vi "MM9.InitDelays.vi"(0 "i ref in":refnum<vi>, 2 "InitObjs":string[](array[string]), 3 "ms timeout (10000)":i32=10000, 5 "error in (no error)":errorcluster) -> (14 "i ref out":refnum<vi>, 16 "InitObjs out":string[](array[string]), 17 "timed out":bool, 19 "error out":errorcluster)   [LabVIEW 2014, in "MM9.lvlib"]
doc: "Initializes the delays."
uses:
  MM9.lvlib
  CSCore/CSSystem/CoreDefs/CoreDefs.call_type.ctl
  CSCore/BaseProcess/BaseProcess.descriptor string definition.ctl
  CSCore/CSSystem/CoreDefs/CoreDefs.rawDataType.ctl
  CSCore/CSSystem/CoreLib/CoreLib.double 2 byte array.vi
  CSCore/BaseProcess/BaseProcess.lvlib
  LEBITLib/LEBITLib.lvlib
  CSCore/CSSystem/CoreLib/CoreLib.lvlib
panel:
  in  "CallClusterTyp":T1={"Object"="", "Selector"="", "CallType"=enum."synchronous", "Async Object"="", "Async Selector"="", "Data Descriptor"="", "Data"=[], "Error #"=0, "Expire"=0}
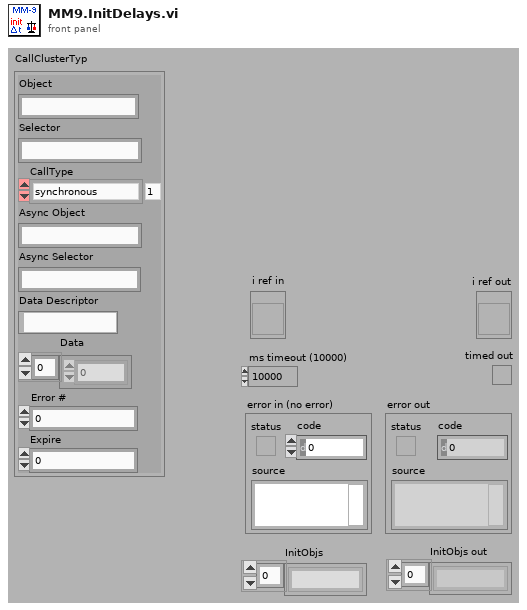
[diagram p1: front panel]
types:
  T1 = typedef "CoreDefs.call_type.ctl" = cluster{"Object":string, "Selector":string, "CallType":enum16{"simple", "synchronous", "asynchronous"}, "Async Object":string, "Async Selector":string, "Data Descriptor":T2, "Data":T3, "Error #":i32, "Expire":u32}
  T2 = typedef "BaseProcess.lvlib/BaseProcess.descriptor string definition.ctl" = string
  T3 = typedef "CoreDefs.rawDataType.ctl" = i8[]
  T4 = enum16{"simple", "synchronous", "asynchronous", "notification"}
  T5 = typedef "MM9.lvlib/MM9.i attribute.ctl" = cluster{"UsedObjs":string[], "ActScanStep":i32[], "AbortRequest":bool, "StopRequest":bool, "# cycles":i32, "Connected":bool, "MMStatus":T6, "# data":i32, "DIMServices":cluster{"MM6StatusString":string, "MM6StatusID":i32, "discArchiver":string, "discArchiverID":i32, "eventBuilder":string, "eventBuilderID":i32, "GUIIDString":string, "GUIIDStringID":i32}, "dataFile":string, "PGRunning":T7, "ConfigData":T8, "ExtraDataSets":T23}
  T6 = typedef "MM9.lvlib/MM9.status.ctl" = enum16{"loaded", "load_error", "config", "config_error", "init", "init_error", "data_reset", "data_reset_error", "running", "start_error", "run_error", "abort_requested", "aborted", "stop_requested", "stopped", "stop_error", "Connected", "NOTConnected"}
  T7 = typedef "PPG_ABC.lvlib/PPG_ABC.PG_Running.ctl" = i32
  T8 = typedef "LEBITDefs9.lvlib/LEBITDefs.ConfigData.ctl" = cluster{"GenConfig":T9, "Configs":T11[]}
  T9 = typedef "LEBITDefs9.lvlib/LEBITDefs.GenConfig.ctl" = cluster{"Mode":i32, "Logs":T10[]}
  T10 = typedef "LEBITDefs9.lvlib/LEBITDefs.Log.ctl" = cluster{"Name":string, "FctName":string, "Special":string}
  T11 = typedef "LEBITDefs9.lvlib/LEBITDefs.OneConfig.ctl" = cluster{"MCA":T12, "Timing":T13, "Scans":T16[], "FreqDevs":T17[], "CleanDev":T18, "NrCycles":i32, "Specials":T20[], "Delays":T21[], "DAC":T22}
  T12 = typedef "LEBITDefs9.lvlib/LEBITDefs.MCA.ctl" = cluster{"Name":string, "Address":string, "NrChannels":i32, "Gate":i32, "NrPipse":i32, "AcqDelay":i32}
  T13 = typedef "LEBITDefs9.lvlib/LEBITDefs.Timing.ctl" = cluster{"TimeTables":cluster{"TimeTable":T14}[], "Memories":T15[], "ScanX":string, "ScanY":string}
  T14 = typedef "LEBITDefs9.lvlib/LEBITDefs.Timetable.ctl" = dbl[]
  T15 = typedef "LEBITDefs9.lvlib/LEBITDefs.Memory.ctl" = cluster{"Device":string, "ExtTrig":bool, "TT2Use":i32, "PatternTable":string[]}
  T16 = typedef "LEBITDefs9.lvlib/LEBITDefs.ScanDev.ctl" = cluster{"Name":string, "FctName":string, "Values":dbl[], "NrScanVals":i32, "Special":string}
  T17 = typedef "LEBITDefs9.lvlib/LEBITDefs.FreqDev.ctl" = cluster{"Name":string, "Amp":dbl, "CenterFreq":dbl, "Time":dbl}
  T18 = typedef "LEBITDefs9.lvlib/LEBITDefs.CleanDev.ctl" = cluster{"Name":string, "CleanData":T19[]}
  T19 = typedef "LEBITDefs9.lvlib/LEBITDefs.CleanDataType.ctl" = cluster{"Amp":dbl, "Center":dbl, "Plus":dbl, "Minus":dbl, "Time":dbl}
  T20 = typedef "LEBITDefs9.lvlib/LEBITDefs.Special.ctl" = cluster{"Name":string, "FctName":string, "VerySpecial":string, "Data":dbl}
  T21 = typedef "LEBITDefs9.lvlib/LEBITDefs.Delay.ctl" = cluster{"Name":string, "Delay":dbl}
  T22 = typedef "LEBITDefs9.lvlib/LEBITDefs.DAC.ctl" = cluster{"Name":string, "Step1":i32, "Step2":i32}
  T23 = typedef "LEBITDefs9.lvlib/LEBITDefs.ExtraData.ctl" = cluster{"Ions":cluster{"ExcitIonMass":string, "ExcitIonCharge":i32, "CleanIons":cluster{"CleanIonMass":string, "CleanIonCharge":i32}[]}, "TimingDescription":cluster{"TimeTableDescription":cluster{"Times":string[]}[], "PatternTableDescription":cluster{"Pattern":string[]}[]}, "ScanUnits":string[]}[]
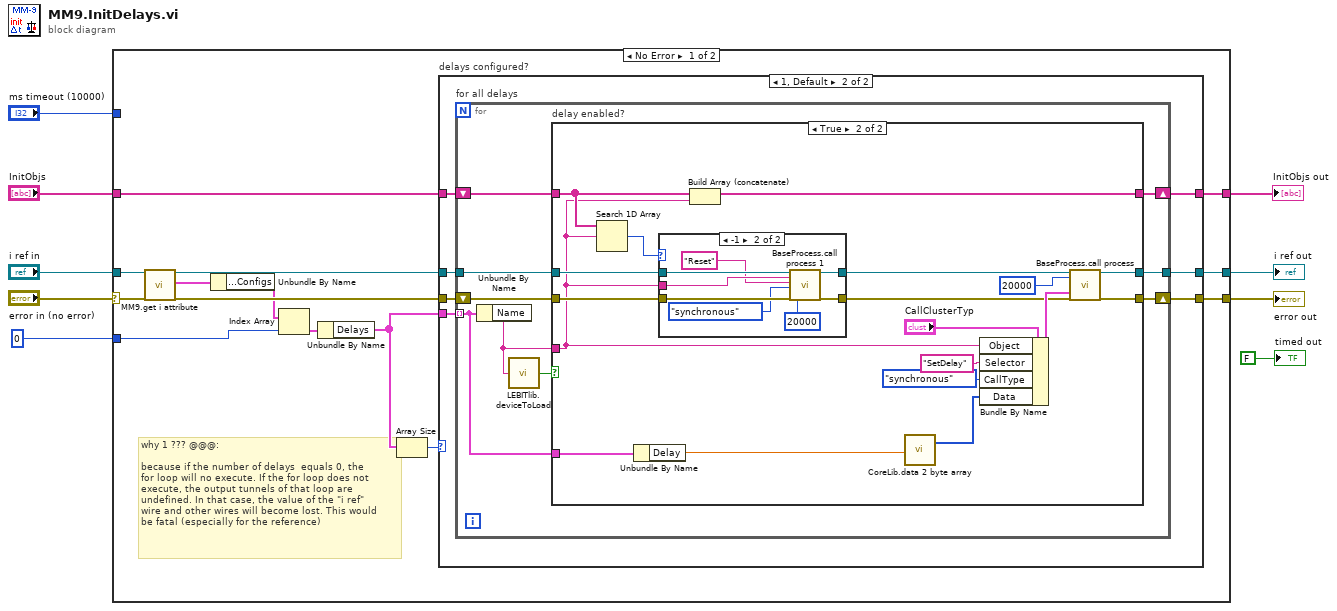
[diagram p0: block diagram]
diagram:
  n1 = case shown="No Error" "error in (no error)" {
    selector: "error in (no error)" -> [w14 w74]
    tunnel: "i ref in" -> [w19 w75]
    tunnel: [w18 w75] -> w8
    tunnel: [w17 w74] -> w7
    tunnel: "InitObjs" -> [w16 w76]
    tunnel: [w15 w76] -> w4
    tunnel: 0 ("index") -> [w10 _]
    tunnel: "ms timeout (10000)" -> [_ _]
    frame No Error {
      # "why 1 ??? @@@:\n\nbecause if the number of delays  equals 0, the \nfor loop will no execute. If the for loop does not\nexecute, the output tunnels of that loop are\nundefined. In that case, the value of the \"i ref\" \nwire and other wires will become lost. This would\nbe fatal (especially for the reference)"
      n2 = call "MM9.get i attribute.vi"("i ref in"=w19, "error in (no error)"=w14) -> ("i ref out"=w21:refnum<vi>, "i attribute"=w13:T5, "error out"=w20:errorcluster)  [unwired: 15 in]
      n3 = Unbundle By Name(w13) -> ("ConfigData.Configs"=w12:T11[])
      n4 = Index Array(array=w12, index=w10) -> (element=w11:T11)
      n5 = Unbundle By Name(w11) -> ("Delays"=w22:T21[])
      n6 = Array Size(array=w22) -> (size(s)=w23:i32)
      n7 = case "delays configured?" shown="1, Default" w23 {
        tunnel: w22 -> [_ w33]
        tunnel: w21 -> [w26 w32]
        tunnel: [w26 w31] -> w18
        tunnel: w20 -> [w25 w27]
        tunnel: [w25 w28] -> w17
        tunnel: w16 -> [w24 w30]
        tunnel: [w24 w29] -> w15
        frame 0 {
        }
        frame 1, Default {
          n8 = for "for all delays" {
            tunnel: w33 -> [w40] mode=indexing
            tunnel: w32 -> [w42]
            tunnel: [w41] -> w31
            shift-right: [w39] -> w29
            shift-left: w30 -> [w38]
            shift-right: [w37] -> w28
            shift-left: w27 -> [w36]
            n9 = Unbundle By Name(w40) -> ("Name"=w34:string)
            n10 = call "LEBITlib.deviceToLoad.vi"("DeviceName"=w34) -> ("DeviceIsToLoad"=w35:bool)
            n11 = case "delay enabled?" shown="True" w35 {
              tunnel: w42 -> [w45 w55]
              tunnel: [w45 w59] -> w41
              tunnel: w36 -> [w44 w54]
              tunnel: w34 -> [_ w49]
              tunnel: [w44 w58] -> w37
              tunnel: w40 -> [_ w63]
              tunnel: w38 -> [w43 w50]
              tunnel: [w43 w48] -> w39
              frame False {
              }
              frame True {
                n12 = Search 1D Array(1D array=w50, element=w49) -> (index of element=w51:i32)  [unwired: 1 in]
                n13 = Unbundle By Name(w63) -> ("Delay"=w46:dbl)
                n14 = case shown="-1" w51 {
                  tunnel: w55 -> [w65 w73]
                  tunnel: w54 -> [w64 w72]
                  tunnel: [w65 w71] -> w53
                  tunnel: [w64 w70] -> w52
                  tunnel: w49 -> [_ w68]
                  frame 0, Default {
                  }
                  frame -1 {
                    n15 = call "BaseProcess.call process 1.vi"("i ref in"=w73, "Object"=w68, "Selector"="Reset", "CallType"=T4."synchronous", "error in (no error)"=w72, "timeout (ms)"=20000) -> ("i ref out"=w71:refnum<vi>, "error out"=w70:errorcluster)  [unwired: 11 in, 1 out]
                  }
                }
                n16 = Build Array (concatenate)(w50, w49) -> (w48:string[])
                n17 = call-poly "CoreLib.data 2 byte array.vi"("f64"=w46) -> ("byteArray out"=w47:T3)  [unwired: 18 in]
                n18 = Bundle By Name(cluster="CallClusterTyp", "Object"=w49, "Selector"="SetDelay", "CallType"=enum16{"simple", "synchronous", "asynchronous"}."synchronous", "Data"=w47) -> (w62:T1)
                n19 = call "BaseProcess.call process.vi"("i ref in"=w53, "timeout (ms)"=20000, "call cluster in"=w62, "error in (no error)"=w52) -> ("i ref out"=w59:refnum<vi>, "error out"=w58:errorcluster)  [unwired: 13 in, 1 out]
              }
            }
          }
        }
      }
    }
    frame Error {
    }
  }
  "error out" <- w7
  "i ref out" <- w8
  "InitObjs out" <- w4
  "timed out" <- FALSE ("timed out")
